vi "Global_linker_path_logger.vi"() -> ()   [LabVIEW 2017]
panel:
  in  "LK_logger":path=path "C:/BD_Monitor/LK__logger.udl"
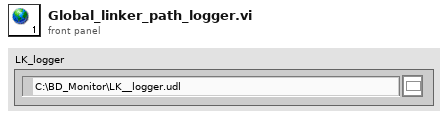
[diagram p1: front panel]
diagram:
